vi "_Main.vi"   [LabVIEW 2017, in "Arm.lvlib"]
uses:
  Arm.lvlib
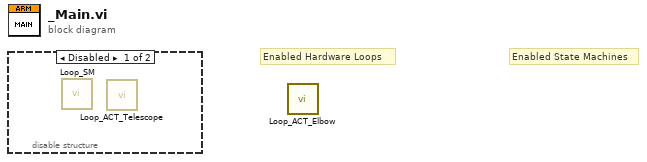
[diagram p0: block diagram]
diagram:
  # "Enabled State Machines"
  # "Enabled Hardware Loops"
  n1 = disable-structure shown="Disabled" {
    frame Disabled {
      n2 = call "Loop_SM.vi"() -> ()  [unwired: 12 in]
      n3 = call "Loop_ACT_Telescope.vi"() -> ()  [unwired: 12 in]
    }
    frame Enabled {
    }
  }
  n4 = call "Loop_ACT_Elbow.vi"() -> ()  [unwired: 12 in]
